vi "XMLPublishStructure.vi"(8 "Error In":errorcluster, 10 "OPC UA server refnum in":refnum<k21>, 11 "DOM document in":refnum<k20>) -> (0 "Error Out":errorcluster, 2 "OPC UA server refnum out":refnum<k21>, 3 "DOM document out":refnum<k20>)   [LabVIEW 2014, in "OPCUA XML(dev).lvlib"]
uses:
  OPCUA XML(dev).lvlib
  <resource>/objmgr/DOMUserDefRef.rc
  <vilib>/xml/NI_XML.lvlib
  <vilib>/xml/Close Reference(Node).vi
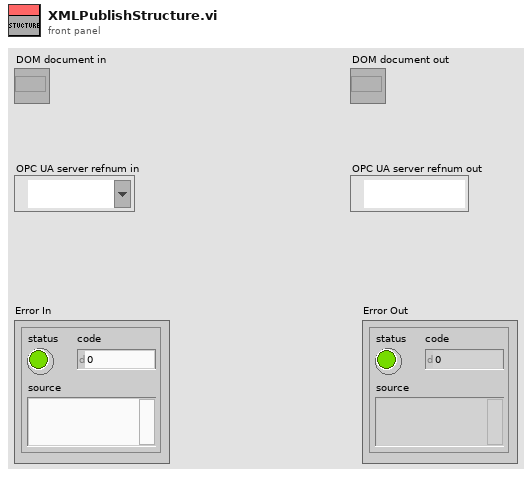
[diagram p1: front panel]
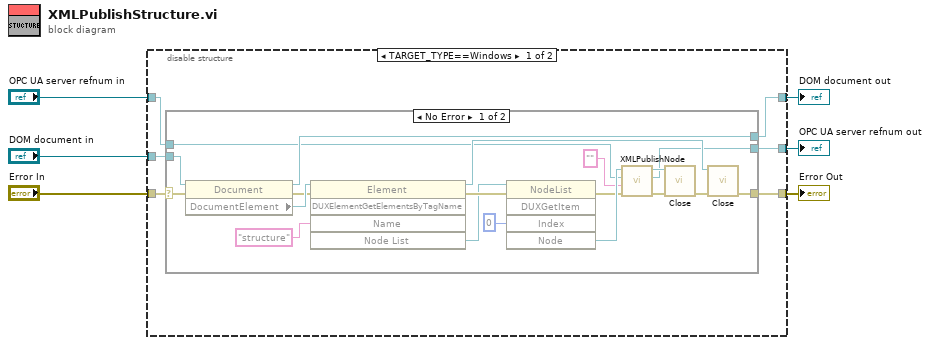
[diagram p0: block diagram]
diagram:
  n1 = disable-structure shown="TARGET_TYPE==Windows" {
    disable-tunnel: [w12 w37] -> w6
    disable-tunnel: "Error In" -> [w11 w37]
    disable-tunnel: "DOM document in" -> [w10 w35]
    disable-tunnel: [w9 w35] -> w3
    disable-tunnel: "OPC UA server refnum in" -> [w8 w36]
    disable-tunnel: [w7 w36] -> w1
    frame condition #0 {
      n2 = case shown="No Error" w11 {
        selector: w11 -> [w31 w34]
        tunnel: [w26 w34] -> w12
        tunnel: w10 -> [w30 w33]
        tunnel: [w29 w33] -> w9
        tunnel: w8 -> [w14 w32]
        tunnel: [w13 w32] -> w7
        frame No Error {
          n3 = property class="Document"(reference=w30, error in=w31) -> (reference out=w29:refnum<k20>, error out=w27:errorcluster, "DocumentElement"=w28:refnum<k20>)
          n4 = invoke class="Element" method="DUXElementGetElementsByTagName"(reference=w28, error in=w27, "Name"="structure") -> (reference out=w22:refnum<k20>, error out=w24:errorcluster, "Node List"=w21:refnum<k20>)  [unwired: 2 in, 2 out]
          n5 = invoke class="NodeList" method="DUXGetItem"(reference=w21, error in=w24, "Index"=0) -> (error out=w19:errorcluster, "Node"=w20:refnum<k20>)  [unwired: 2 in, 3 out]
          n6 = call "XMLPublishNode.vi"("Error In"=w19, "parent opcua path"="", "OPC UA server refnum in"=w14, "DOM node"=w20) -> ("Error Out"=w16:errorcluster, "OPC UA server refnum out"=w13:refnum<k21>, "DOM node (dup)"=w17:refnum<k20>)  [unwired: 5 in]
          n7 = call-poly <vilib>:"Close.vi"("error in (no error)"=w16, "node"=w17) -> ("error out"=w15:errorcluster)  [unwired: 7 out]
          n8 = call-poly <vilib>:"Close.vi"("error in (no error)"=w15, "node"=w22) -> ("error out"=w26:errorcluster)  [unwired: 7 out]
        }
        frame Error {
        }
      }
    }
    frame condition #1 (active) {
    }
  }
  "Error Out" <- w6
  "DOM document out" <- w3
  "OPC UA server refnum out" <- w1
